vi "AnalyzeBlobs.vi"(9 "Vision Target":enum16{"Pegs", "Gears"}(ring), 10 "Blob Data":T1, 11 "Image In":T2) -> (2 "Target Data":cluster{"X":dbl, "Distance":dbl}, 3 "Image Out":T2)   [LabVIEW 2016]
uses:
  <vilib>/vision/Image Controls.llb/IMAQ Image.ctl
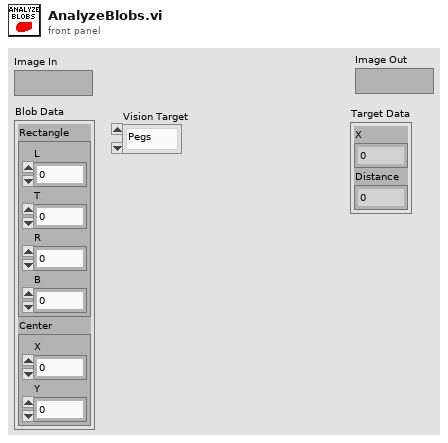
[diagram p1: front panel]
types:
  T1 = cluster{"Rectangle":cluster{"L":dbl, "T":dbl, "R":dbl, "B":dbl}, "Center":cluster{"X":dbl, "Y":dbl}}
  T2 = typedef "IMAQ Image.ctl" = refnum<image>
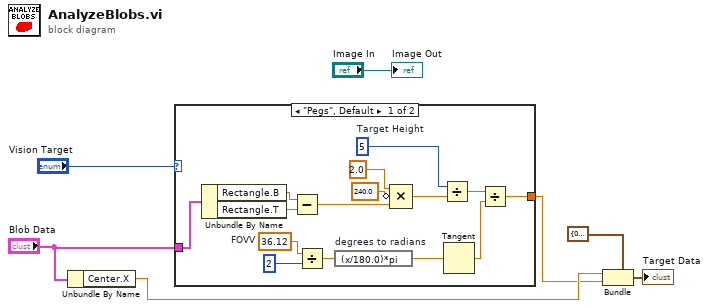
[diagram p0: block diagram]
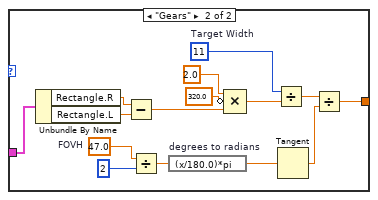
[diagram p2: hidden frame]
diagram:
  n1 = Unbundle By Name("Blob Data") -> ("Center.X"=w5:dbl)
  n2 = case shown="\"Pegs\", Default" "Vision Target" {
    tunnel: "Blob Data" -> [w9 w24]
    tunnel: [w8 w23] -> w4
    frame "Pegs", Default {
      w18 = 36.12  # FOVV
      w11 = 5  # Target Height
      n3 = Unbundle By Name(w9) -> ("Rectangle.B"=w16:dbl, "Rectangle.T"=w15:dbl)
      n4 = Subtract(x=w16, y=w15) -> (x-y=w17:dbl)
      n5 = Divide(x=w18, y=2) -> (x/y=w21:dbl)
      n6 = expression code="(x/180.0)*pi" "degrees to radians"(w21) -> (w22:dbl)
      n7 = Compound Arithmetic op=MULTIPLY(2.0, invert 240.0 ("value"), w17) -> (w13:dbl)
      n8 = Divide(x=w11, y=w13) -> (x/y=w20:dbl)
      n9 = Tangent(1:w22) -> (0:w10:dbl)
      n10 = Divide(x=w20, y=w10) -> (x/y=w8:dbl)
    }
    frame "Gears" {
      w33 = 47.0  # FOVH
      w26 = 11  # Target Width
      n11 = Unbundle By Name(w24) -> ("Rectangle.R"=w31:dbl, "Rectangle.L"=w30:dbl)
      n12 = Subtract(x=w31, y=w30) -> (x-y=w32:dbl)
      n13 = Divide(x=w33, y=2) -> (x/y=w36:dbl)
      n14 = expression code="(x/180.0)*pi" "degrees to radians"(w36) -> (w37:dbl)
      n15 = Compound Arithmetic op=MULTIPLY(2.0, invert 320.0 ("value"), w32) -> (w28:dbl)
      n16 = Divide(x=w26, y=w28) -> (x/y=w35:dbl)
      n17 = Tangent(1:w37) -> (0:w25:dbl)
      n18 = Divide(x=w35, y=w25) -> (x/y=w23:dbl)
    }
  }
  n19 = Bundle(cluster=cluster{"X":dbl, "Distance":dbl} {"X"=0.0, "Distance"=0.0}, "X"=w5, "Distance"=w4) -> (→"Target Data":cluster{"X":dbl, "Distance":dbl})
  "Image Out" <- "Image In"
